vi "LidarSetup.vi"() -> ()   [LabVIEW 2024]
uses:
  e33ea129-5426-40bd-9da2-e127971607b1.vi
  <vilib>/Instr/_visa.llb/VISA Configure Serial Port (Instr).vi
  <vilib>/Python/Open Venv Python Session.vi
panel:
  in  "min smaples":i32
  in  "eps":i32
  out "y_array":i32[](array[numeric])
  out "x_array":i32[](array[numeric])
  out "error out":errorcluster
  out "Python Loop Process Time":u32=101
  in  "Tab Control":enum32{"Lidar", "Buffer"}(tab)
  out "LiDAR_ROI":cluster{i32[], i32[]}(graph)
  in  "COM4 2":refnum<visa-resource-name>="COM3" caption="LiDAR_Com."
  in  "격자크기":dbl=20.0
  in  "Stop":bool
  out "Loop Time":u32=102
  out "read buffer":string
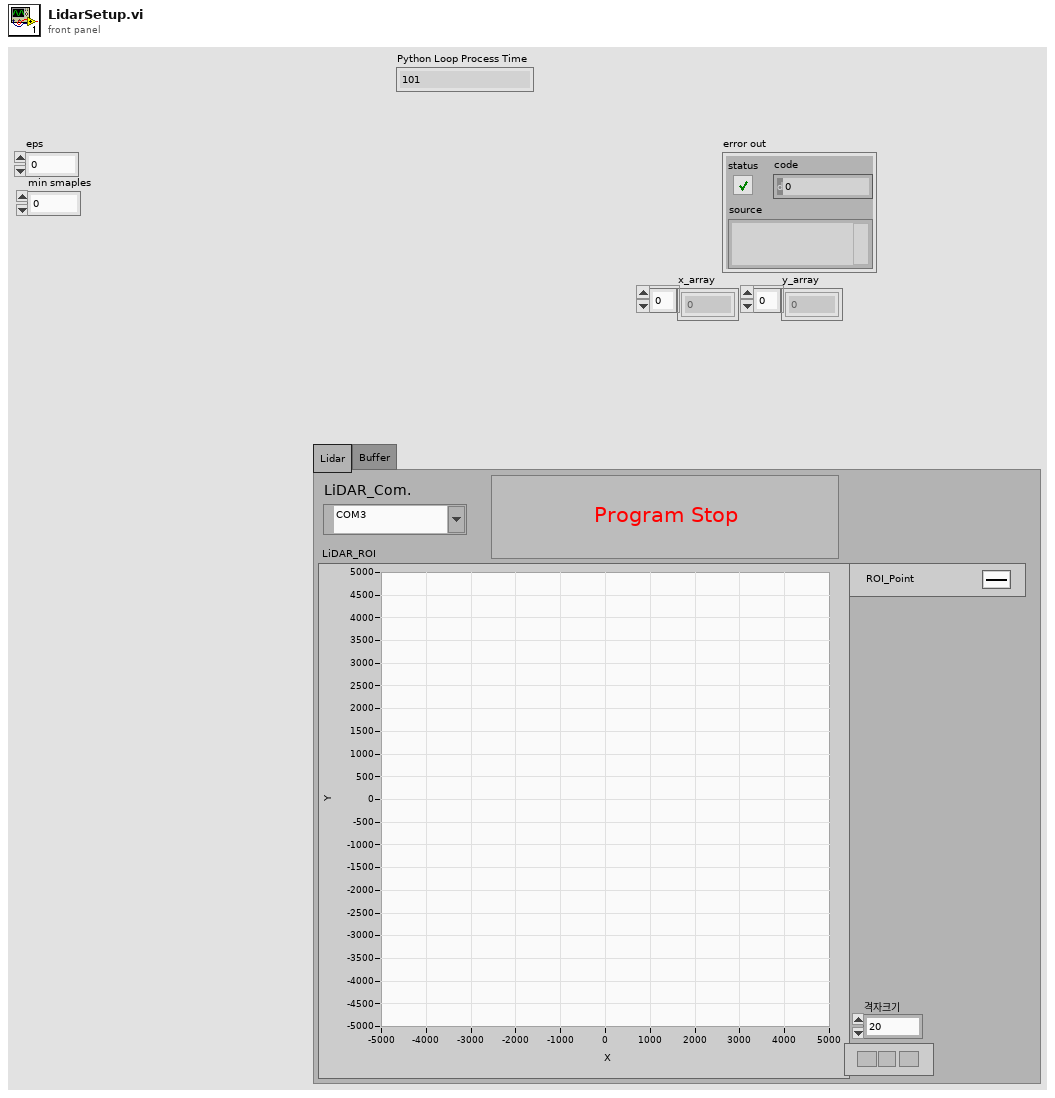
[diagram p1: front panel]
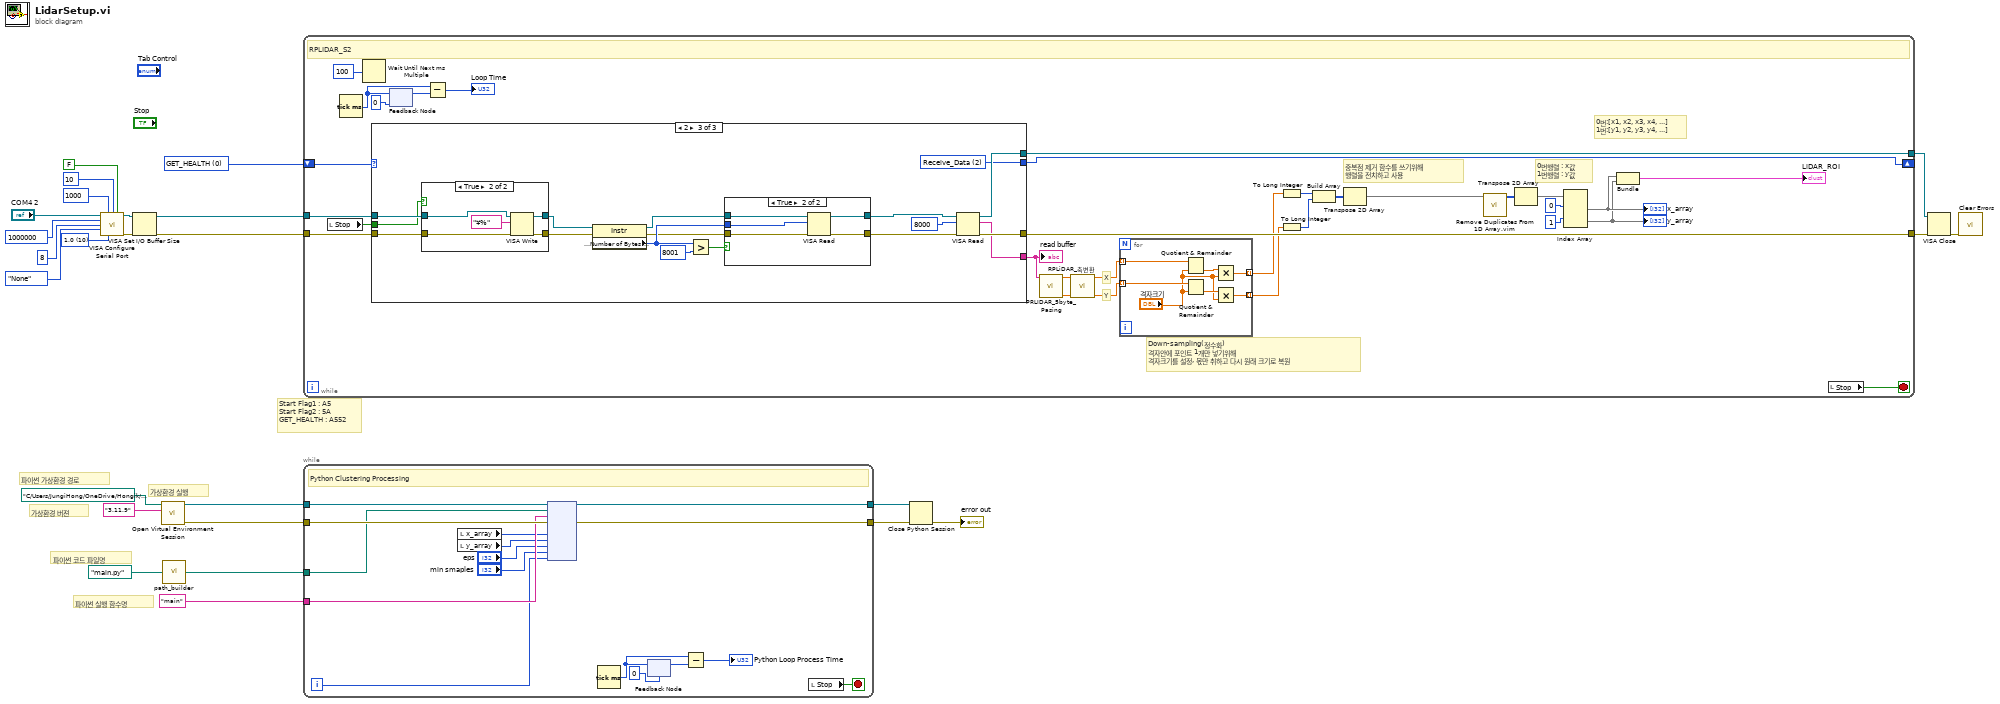
[diagram p0: block diagram]
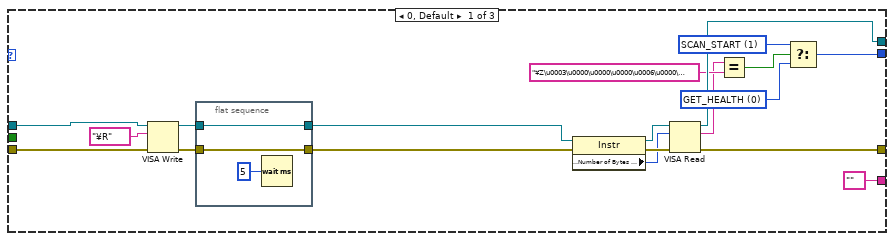
[diagram p2: hidden frame]
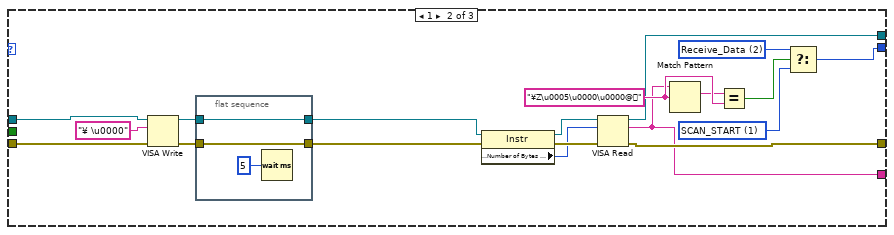
[diagram p3: hidden frame]
diagram:
  w11 = u16 10 items=["1.0"=10, "1.5"=15, "2.0"=20] ("stop bits (10: 1 bit)")
  w13 = u16 0 items=["GET_HEALTH", "SCAN_START", "Receive_Data"]
  # "파이썬 실행 함수명"
  # "파이썬 코드 파일명"
  # "가상환경 실행"
  # "가상환경 버젼"
  # "파이썬 가상환경 경로"
  # "Start Flag1 : A5\nStart Flag2 : 5A \nGET_HEALTH : A552"
  n1 = call-poly "VISA Configure Serial Port"("VISA resource name"="COM4 2", "timeout (10sec)"=u32 1000, "termination char\n(0xA = '\\n' = LF)"=u8 10 ("termination char\n(0xA = '\\n' = LF)"), "Enable Termination\nChar (T)"=FALSE ("Enable Termination\nChar (T)"), "baud rate (9600)"=u32 1000000, "data bits (8)"=u16 8, "parity (0:none)"=enum16{"None", "Odd", "Even", "Mark", "Space"}."None", "stop bits (10: 1 bit)"=w11) -> ("VISA resource name out"=w21:refnum<visa-resource-name>, "error out"=w20:errorcluster)  [unwired: 6 in]
  n2 = VISA Set I/O Buffer Size(VISA resource name=w21, error in (no error)=w20) -> (VISA resource name out=w15:refnum<visa-resource-name>, error out=w14:errorcluster)  [unwired: 2 in]
  n3 = call-poly <vilib>:"Open Virtual Environment Session.vi"("Python version"="3.11.9", "Env path"=path "C:/Users/JungiHong/OneDrive/Hongik/HI-RACE/2026-01/.venv") -> ("error out"=w5:errorcluster, "session out"=w6:refnum<k35>)  [unwired: 8 in]
  n4 = call "path_builder.vi"("Name"=path "main.py") -> ("appended path"=w4:path)
  n5 = while {
    tunnel: [w47] -> w25
    tunnel: [w48] -> w24
    tunnel: w15 -> [w56]
    tunnel: w14 -> [w55]
    shift-right: [w54] -> _
    shift-left: w13 -> [w57]
    stop <- w30 stop-if-true
    # "0번:[x1, x2, x3, x4, ...]\n1번:[y1, y2, y3, y4, ...]"
    # "0번행렬 : x값\n1번행렬 : y값"
    # "중복점 제거 함수를 쓰기위해\n행렬을 전치하고 사용"
    # "Down-sampling(정수화)\n격자안에 포인트 1개만 넣기위해\n격자크기를 설정, 몫만 취하고 다시 원래 크기로 복원"
    # "Y"
    # "X"
    # "RPLIDAR_S2"
    n6 = local read "Stop"() -> (w53:bool)
    n7 = Tick Count (ms)() -> (millisecond timer value=w52:u32)
    n8 = Wait Until Next ms Multiple(millisecond multiple=u32 100 ("ms 배수")) -> ()  [unwired: 1 out]
    n9 = case shown="2" w57 {
      tunnel: w56 -> [w82 w100 w123]
      tunnel: w55 -> [w81 w99 w122]
      tunnel: [w83 w96 w109] -> w54
      tunnel: [w72 w97 w125] -> w48
      tunnel: [w71 w98 w124] -> w47
      tunnel: w53 -> [_ _ w121]
      tunnel: ["" ("read buffer") w94 w120] -> w31
      frame 0, Default {
        w65 = u16 0 items=["GET_HEALTH", "SCAN_START", "Receive_Data"]
        w66 = u16 1 items=["GET_HEALTH", "SCAN_START", "Receive_Data"]
        n10 = VISA Write(VISA resource name=w82, write buffer="¥R", error in (no error)=w81) -> (VISA resource name out=w76:refnum<visa-resource-name>, error out=w75:errorcluster)  [unwired: 1 out]
        n11 = flat-sequence {
          tunnel: w76 -> [w85]
          tunnel: w75 -> [w84]
          tunnel: [w85] -> w74
          tunnel: [w84] -> w73
          frame #0 {
            n12 = Wait (ms)(milliseconds to wait=u32 5 ("대기 시간 (ms)")) -> ()  [unwired: 1 out]
          }
        }
        n13 = property class="Instr"(reference=w74, error in=w73) -> (reference out=w79:refnum<visa-resource-name>, error out=w78:errorcluster, "Serial Settings:Number of Bytes at Serial Port"=w77:u32)
        n14 = VISA Read(VISA resource name=w79, byte count=w77, error in (no error)=w78) -> (VISA resource name out=w71:refnum<visa-resource-name>, read buffer=w68:string, error out=w72:errorcluster)  [unwired: 1 out]
        n15 = Equal?(x=w68, y="¥Z\u0003\u0000\u0000\u0000\u0006\u0000\u0000\u0000") -> (x = y?=w69:bool)
        n16 = Select(t=w66, s=w69, f=w65) -> (s? t:f=w83:u16)
      }
      frame 1 {
        w87 = u16 2 items=["GET_HEALTH", "SCAN_START", "Receive_Data"]
        w88 = u16 1 items=["GET_HEALTH", "SCAN_START", "Receive_Data"]
        w101 = "¥Z\u0005\u0000\u0000@"
        n17 = VISA Write(VISA resource name=w100, write buffer="¥ \u0000", error in (no error)=w99) -> (VISA resource name out=w103:refnum<visa-resource-name>, error out=w104:errorcluster)  [unwired: 1 out]
        n18 = flat-sequence {
          tunnel: w103 -> [w107]
          tunnel: w104 -> [w106]
          tunnel: [w107] -> w90
          tunnel: [w106] -> w89
          frame #0 {
            n19 = Wait (ms)(milliseconds to wait=u32 5 ("대기 시간 (ms)")) -> ()  [unwired: 1 out]
          }
        }
        n20 = property class="Instr"(reference=w90, error in=w89) -> (reference out=w93:refnum<visa-resource-name>, error out=w92:errorcluster, "Serial Settings:Number of Bytes at Serial Port"=w91:u32)
        n21 = VISA Read(VISA resource name=w93, byte count=w91, error in (no error)=w92) -> (VISA resource name out=w98:refnum<visa-resource-name>, read buffer=w94:string, error out=w97:errorcluster)  [unwired: 1 out]
        n22 = Match Pattern(string=w94, regular expression=w101) -> (match substring=w95:string)  [unwired: 1 in, 3 out]
        n23 = Equal?(x=w95, y=w101) -> (x = y?=w105:bool)
        n24 = Select(t=w87, s=w105, f=w88) -> (s? t:f=w96:u16)
      }
      frame 2 {
        w109 = u16 2 items=["GET_HEALTH", "SCAN_START", "Receive_Data"]
        n25 = case shown="True" w121 {
          tunnel: w123 -> [w134 w138]
          tunnel: w122 -> [w133 w137]
          tunnel: [w134 w136] -> w119
          tunnel: [w133 w135] -> w118
          frame False {
          }
          frame True {
            n26 = VISA Write(VISA resource name=w138, write buffer="¥%", error in (no error)=w137) -> (VISA resource name out=w136:refnum<visa-resource-name>, error out=w135:errorcluster)  [unwired: 1 out]
          }
        }
        n27 = property class="Instr"(reference=w119, error in=w118) -> (reference out=w114:refnum<visa-resource-name>, error out=w113:errorcluster, "Serial Settings:Number of Bytes at Serial Port"=w115:u32)
        n28 = Greater?(x=w115, y=u32 8001) -> (0:w117:bool)
        n29 = case shown="True" w117 {
          tunnel: w114 -> [w127 w132]
          tunnel: w115 -> [_ w131]
          tunnel: w113 -> [w126 w130]
          tunnel: [w127 w129] -> w112
          tunnel: [w126 w128] -> w111
          frame False {
          }
          frame True {
            n30 = VISA Read(VISA resource name=w132, byte count=w131, error in (no error)=w130) -> (VISA resource name out=w129:refnum<visa-resource-name>, error out=w128:errorcluster)  [unwired: 2 out]
          }
        }
        n31 = VISA Read(VISA resource name=w112, byte count=u32 8000, error in (no error)=w111) -> (VISA resource name out=w124:refnum<visa-resource-name>, read buffer=w120:string, error out=w125:errorcluster)  [unwired: 1 out]
      }
    }
    "read buffer" <- w31
    n32 = feedback #1(u32 0 ("millisecond timer value")) -> (w51:u32)
    n33 = feedback-in #1(w52) -> ()
    n34 = Subtract(x=w52, y=w51) -> (x-y=→"Loop Time":u32)
    n35 = call "PRLIDAR_5byte_Pasing.vi"("RPLIDAR_Data"=w31) -> ("Theta(deg)"=w34:dbl[], "Distance(mm)"=w35:dbl[])  [unwired: 9 in]
    n36 = call "RPLiDAR_축변환.vi"("Distance(mm)"=w34, "Theta(deg)"=w35) -> ("Y"=w32:dbl[], "X"=w33:dbl[])  [unwired: 8 in]
    n37 = for {
      tunnel: w33 -> [w64] mode=indexing
      tunnel: w32 -> [w63] mode=indexing
      tunnel: [w60] -> w45 mode=indexing
      tunnel: [w59] -> w46 mode=indexing
      n38 = Quotient & Remainder(x=w64, y="격자크기") -> (floor(x/y)=w62:dbl)  [unwired: 1 out]
      n39 = Quotient & Remainder(x=w63, y="격자크기") -> (floor(x/y)=w61:dbl)  [unwired: 1 out]
      n40 = Multiply(x=w62, y="격자크기") -> (x*y=w60:dbl)
      n41 = Multiply(x=w61, y="격자크기") -> (x*y=w59:dbl)
    }
    n42 = To Long Integer(number=w45) -> (32bit integer=w39:i32[])
    n43 = To Long Integer(number=w46) -> (32bit integer=w38:i32[])
    n44 = Build Array(w39, w38) -> (w41:i32[][])
    n45 = Transpose 2D Array(2D array=w41) -> (transposed array=w36:i32[][])
    n46 = call "Remove Duplicates From 1D Array.vim"("array"=w36) -> ("array with duplicates removed"=w37:i32[][])  [unwired: 10 in]
    n47 = Transpose 2D Array(2D array=w37) -> (transposed array=w42:i32[][])
    n48 = Index Array(array=w42, index (row) #1=0 ("index (row)"), index (row) #2=1 ("index (row)")) -> (element #1=w28:i32[], element #2=w27:i32[])  [unwired: 2 in]
    "x_array" <- w28
    "y_array" <- w27
    n49 = Bundle(w28, w27) -> (→"LiDAR_ROI":cluster{i32[], i32[]})  [unwired: 1 in]
    n50 = local read "Stop"() -> (w30:bool)
  }
  n51 = while {
    tunnel: w4 -> [w151]
    tunnel: "main" ("module out") -> [w150]
    tunnel: w6 -> [w153]
    tunnel: [w155] -> w8
    tunnel: w5 -> [w152]
    tunnel: [w154] -> w7
    i -> [w141]
    stop <- w149 stop-if-true
    # "Python Clustering Processing"
    n52 = local read "x_array"() -> (w144:i32[])
    n53 = local read "y_array"() -> (w143:i32[])
    n54 = node(w153, w151, w150, w152, w144, w143, "eps", "min smaples", w141) -> (w155:refnum<k35>, w154:errorcluster)  [unwired: 7 in, 2 out]
    n55 = Tick Count (ms)() -> (millisecond timer value=w145:u32)
    n56 = feedback #2(u32 0 ("millisecond timer value")) -> (w146:u32)
    n57 = feedback-in #2(w145) -> ()
    n58 = Subtract(x=w145, y=w146) -> (x-y=→"Python Loop Process Time":u32)
    n59 = local read "Stop"() -> (w149:bool)
  }
  n60 = Close Python Session(session in=w8, error in=w7) -> (11:→"error out":errorcluster)
  n61 = VISA Close(VISA resource name=w25, error in (no error)=w24) -> (error out=w26:errorcluster)
  n62 = call <vilib>:"Clear Errors.vi"("error in (no error)"=w26) -> ()  [unwired: 5 in, 2 out]
